vi "STAT2 decode Analog data from Controller.vi"(9 "Temperature base conversion factor":u16, 10 "Controller local":T1 {"High G monitoring" format="%02x"; "NA" format="%02x"; "GPIO values" format="%02x"; "Relay status" format="%02x"; "sys register" format="%04x"}) -> (2 "Controller analog data":dbl[](array[numeric]), 3 "Temperature":dbl)   [LabVIEW 2011]
uses:
  LEINmaster/Nodes/Controller local stat2.ctl
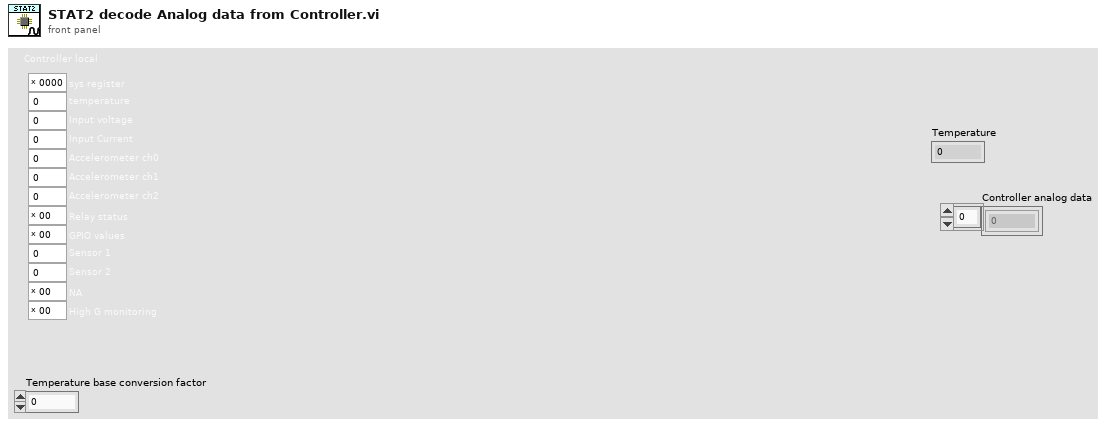
[diagram p1: front panel]
types:
  T1 = typedef "Controller local stat2.ctl" = cluster{"sys register":u16, "temperature":u16, "Input voltage":u16, "Input Current":u16, "Accelerometer ch0":u16, "Accelerometer ch1":u16, "Accelerometer ch2":u16, "Relay status":u8, "GPIO values":u8, "Sensor 1":i32, "Sensor 2":i32, "NA":u8, "High G monitoring":u8}
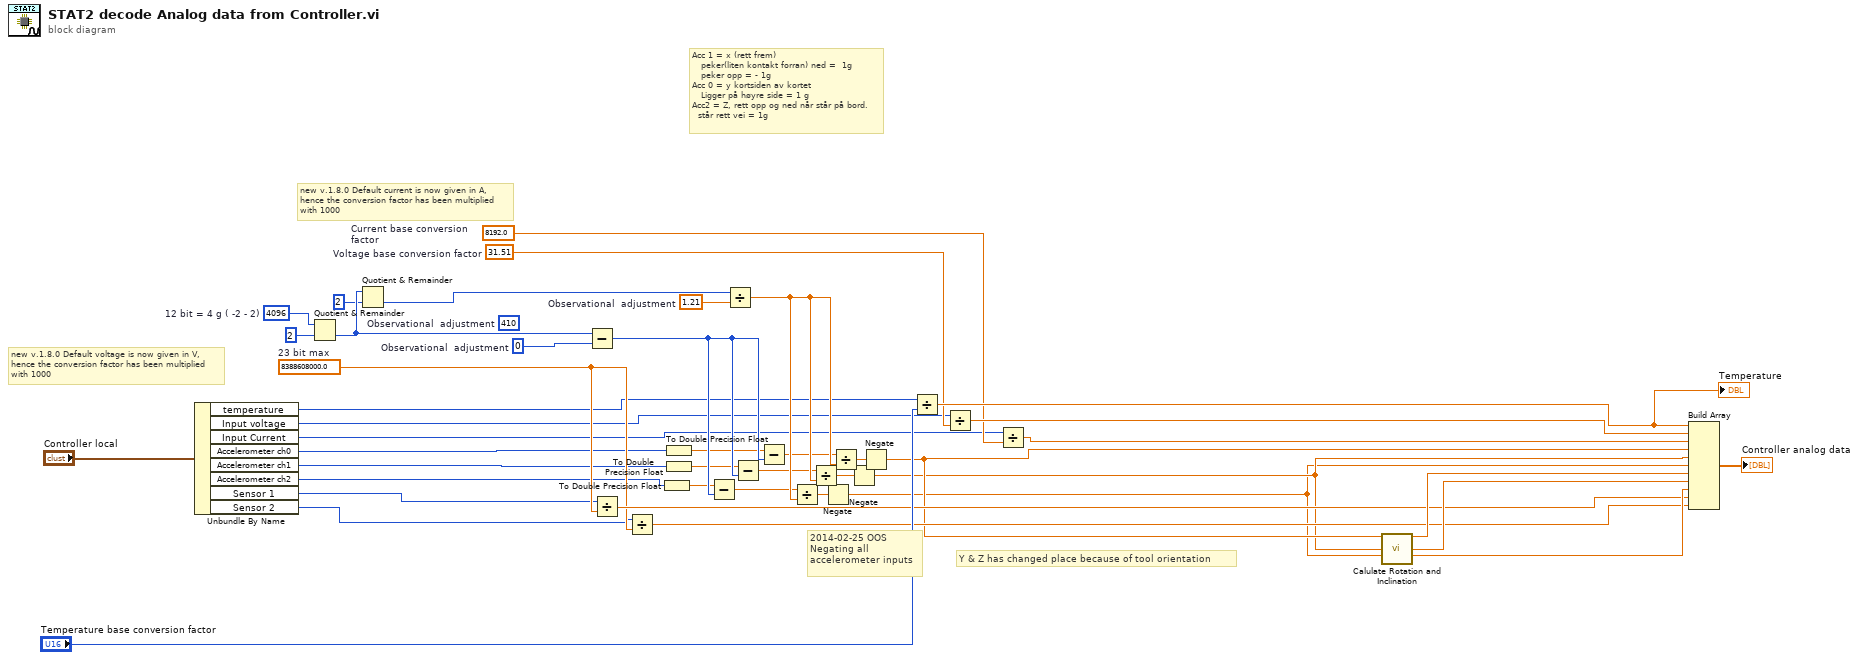
[diagram p0: block diagram]
diagram:
  (unwired) 410  # Observational  adjustment
  w42 = 1.21  # Observational  adjustment
  w33 = 0  # Observational  adjustment
  w26 = 8388608000.0  # 23 bit max
  w10 = 4096  # 12 bit = 4 g ( -2 - 2)
  w9 = 8192.0  # Current base conversion factor
  w7 = 31.51  # Voltage base conversion factor
  # "Y & Z has changed place because of tool orientation"
  # "2014-02-25 OOS\nNegating all \naccelerometer inputs"
  # "new v.1.8.0 Default voltage is now given in V, \nhence the conversion factor has been multiplied\nwith 1000"
  # "new v.1.8.0 Default current is now given in A, \nhence the conversion factor has been multiplied\nwith 1000"
  # "Acc 1 = x (rett frem)\n   peker(liten kontakt forran) ned =  1g\n   peker opp = - 1g\nAcc 0 = y kortsiden av kortet\n   Ligger på høyre side = 1 g\nAcc2 = Z, rett opp og ned når står på bord.\n  står rett vei = 1g"
  n1 = Unbundle By Name("Controller local") -> ("temperature"=w5:u16, "Input voltage"=w6:u16, "Input Current"=w8:u16, "Accelerometer ch0"=w13:u16, "Accelerometer ch1"=w15:u16, "Accelerometer ch2"=w23:u16, "Sensor 1"=w24:i32, "Sensor 2"=w25:i32)
  n2 = Quotient & Remainder(x=w10, y=2) -> (floor(x/y)=w18:i32)  [unwired: 1 out]
  n3 = Quotient & Remainder(x=w18, y=2) -> (floor(x/y)=w22:i32)  [unwired: 1 out]
  n4 = Subtract(x=w18, y=w33) -> (x-y=w32:i32)
  n5 = Divide(x=w24, y=w26) -> (x/y=w30:dbl)
  n6 = Divide(x=w25, y=w26) -> (x/y=w29:dbl)
  n7 = To Double Precision Float(number=w23) -> (double precision float=w16:dbl)
  n8 = To Double Precision Float(number=w13) -> (double precision float=w12:dbl)
  n9 = To Double Precision Float(number=w15) -> (double precision float=w14:dbl)
  n10 = Subtract(x=w16, y=w32) -> (x-y=w21:dbl)
  n11 = Divide(x=w22, y=w42) -> (x/y=w34:dbl)
  n12 = Subtract(x=w14, y=w32) -> (x-y=w20:dbl)
  n13 = Subtract(x=w12, y=w32) -> (x-y=w19:dbl)
  n14 = Divide(x=w21, y=w34) -> (x/y=w36:dbl)
  n15 = Divide(x=w20, y=w34) -> (x/y=w35:dbl)
  n16 = Negate(x=w36) -> (-x=w1:dbl)
  n17 = Divide(x=w19, y=w34) -> (x/y=w37:dbl)
  n18 = Negate(x=w35) -> (-x=w2:dbl)
  n19 = Negate(x=w37) -> (-x=w3:dbl)
  n20 = Divide(x=w5, y="Temperature base conversion factor") -> (x/y=w41:dbl)
  "Temperature" <- w41
  n21 = Divide(x=w6, y=w7) -> (x/y=w27:dbl)
  n22 = Divide(x=w8, y=w9) -> (x/y=w28:dbl)
  n23 = call "Calulate Rotation and Inclination.vi"("Ch 0"=w3, "Ch 1"=w2, "Ch 2"=w1) -> ("Magnitude XYZ(g)"=w39:dbl, "Inclination"=w40:dbl, "Rotation"=w38:dbl)  [unwired: 10 in]
  n24 = Build Array(w41, w27, w28, w3, w2, w1, w39, w40, w38, w30, w29) -> (→"Controller analog data":dbl[])
